vi "Test Failing Dummy Method.vi"(8 "error in (no error)":errorcluster, 11 "Dummy Test Case in":refnum<class "Dummy.lvclass">) -> (0 "error out":errorcluster, 3 "Dummy Test Case out":refnum<class "Dummy.lvclass">)   [LabVIEW 2020, in "Test Finder Test Dummy.lvlib" / "Dummy.lvclass"]
uses:
  Dummy.lvclass
  C:/git/astemes-lunit/source/API/LUnit Test Case/LUnit Test Case.lvclass
  source/API/LUnit Test Case/LUnit Test Case.lvclass/LUnit Test Case.ctl
  source/API/LUnit Test Case/Private/Append Fail Result.vi
  Dummy.lvclass/Dummy.ctl
  source/API/LUnit Test Case/LUnit Test Case.lvclass
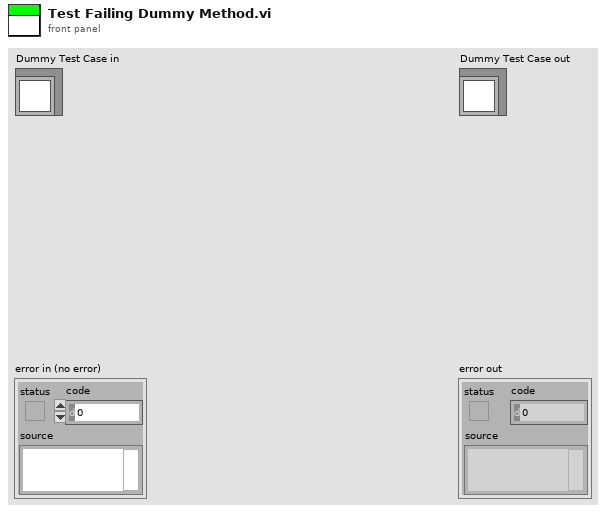
[diagram p1: front panel]
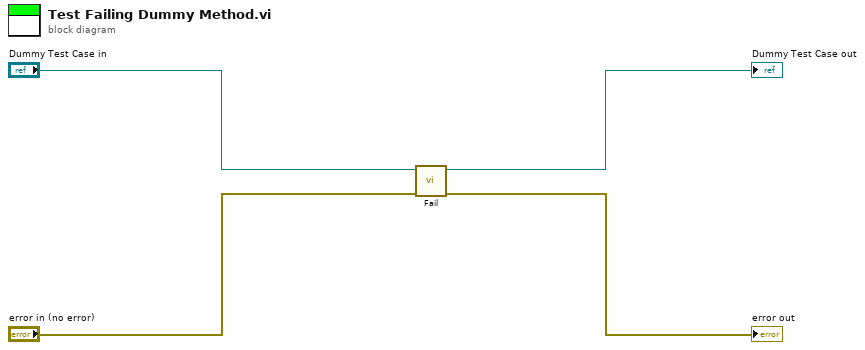
[diagram p0: block diagram]
diagram:
  n1 = call "Fail.vi"("error in (no error)"="error in (no error)", "LUnit Test Case In"="Dummy Test Case in") -> ("error out"=→"error out":errorcluster, "LUnit Test Case Out"=→"Dummy Test Case out":refnum<class "Dummy.lvclass">)  [unwired: 8 in]
